vi "csvtodata.vi"(5 "y軸の列数\ncolumn num\nof y axis":i32=1, 7 "x軸の列数\ncolumn num\nof x axis":i32, 9 "区切り文字\ndelimiter":string="\t", 10 "num of lines to ignore":i32=1, 11 "file path (use dialog)":path) -> (0 "error out":errorcluster, 1 "path":path, 2 "y":dbl[](array[numeric]), 3 "x":dbl[](array[numeric]))   [LabVIEW 2020]
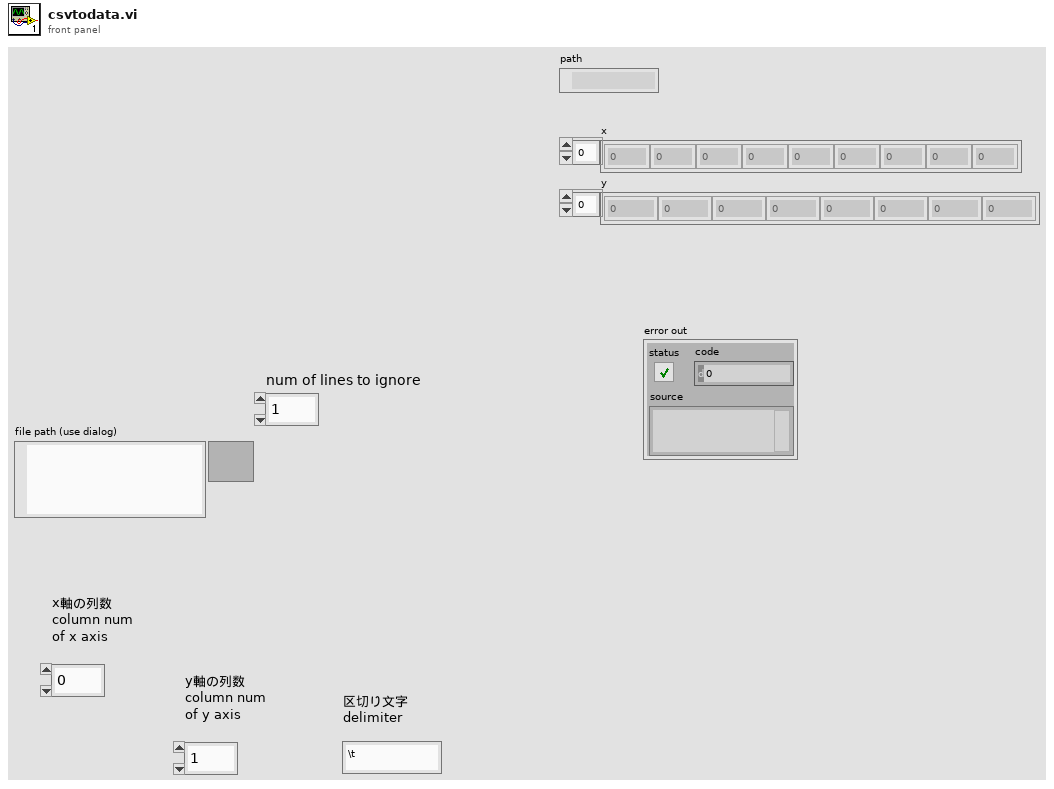
[diagram p1: front panel]
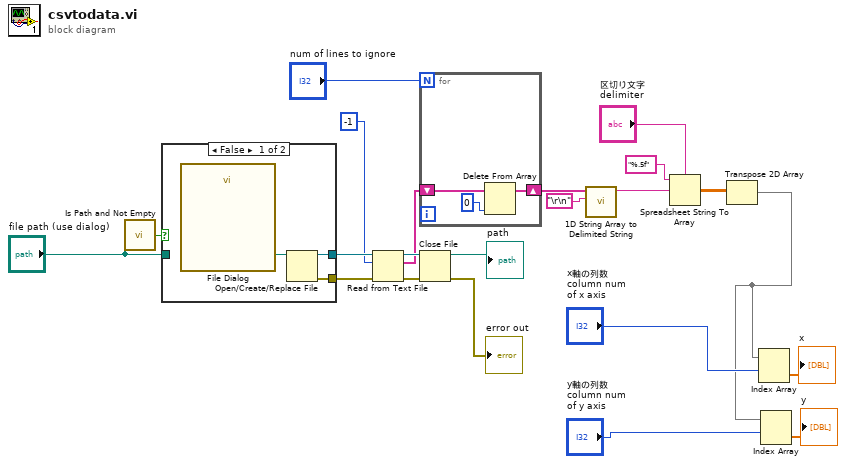
[diagram p0: block diagram]
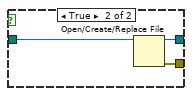
[diagram p2: hidden frame]
diagram:
  n1 = call <vilib>:"Is Path and Not Empty.vi"("path"="file path (use dialog)") -> ("Is Path and Not Empty?"=w22:bool)  [unwired: 4 in]
  n2 = case shown="False" w22 {
    tunnel: "file path (use dialog)" -> [_ w28]
    tunnel: [w24 w27] -> w18
    tunnel: [w23 w26] -> w17
    frame False {
      n3 = call "File Dialog"() -> ("selected path"=w25:path)  [unwired: 12 in, 3 out]
      n4 = Open/Create/Replace File(file path (use dialog)=w25) -> (refnum out=w24:refnum<file>, error out=w23:errorcluster)  [unwired: 5 in, 1 out]
    }
    frame True {
      n5 = Open/Create/Replace File(file path (use dialog)=w28) -> (refnum out=w27:refnum<file>, error out=w26:errorcluster)  [unwired: 5 in, 1 out]
    }
  }
  n6 = Read from Text File(file (use dialog)=w18, count=-1, error in=w17) -> (refnum out=w15:refnum<file>, text=w11:string[], error out=w14:errorcluster)  [unwired: 1 in, 1 out]
  n7 = for {
    N: "num of lines to ignore" -> [_]
    shift-right: [w29] -> w10
    shift-left: w11 -> [w31]
    n8 = Delete From Array(array=w31, index=0) -> (array with subset deleted=w29:string[])  [unwired: 1 in, 1 out]
  }
  n9 = Close File(refnum=w15, error in=w14) -> (path=→"path":path, error out=→"error out":errorcluster)
  n10 = call <vilib>:"1D String Array to Delimited String.vi"("delimiter"="\r\n", "string array"=w10) -> ("delimited string"=w8:string)  [unwired: 9 in]
  n11 = Spreadsheet String To Array(delimiter (Tab)="区切り文字\ndelimiter", format string="%.5f" ("format (%.3f)"), spreadsheet string=w8) -> (array=w6:dbl[][])  [unwired: 1 in]
  n12 = Transpose 2D Array(2D array=w6) -> (transposed array=w4:dbl[][])
  n13 = Index Array(array=w4, index (row)="x軸の列数\ncolumn num\nof x axis") -> (element=→"x":dbl[])  [unwired: 1 in]
  n14 = Index Array(array=w4, index (row)="y軸の列数\ncolumn num\nof y axis") -> (element=→"y":dbl[])  [unwired: 1 in]
